vi "Read Session.vi"(8 "error in":errorcluster, 11 "Fgen PXI in":refnum<class "Fgen PXI.lvclass">) -> (0 "error out":errorcluster, 2 "Session":refnum<k15>, 3 "Fgen PXI out":refnum<class "Fgen PXI.lvclass">)   [LabVIEW 2023, in "Fgen PXI.lvlib" / "Fgen PXI.lvclass"]
uses:
  Fgen PXI.lvclass
  Fgen PXI.lvclass/Fgen PXI.ctl
  Fgen PXI CFG/Fgen PXI CFG.lvclass
  D:/git/HAL/Fgen Base/Fgen Base.lvclass
  D:/git/HAL/Instrument/Instrument.lvclass
  D:/git/HAL/Interfaces/IFGEN/IFGEN.lvclass
  D:/git/HAL/Fgen PXI/Fgen PXI.lvclass
  Fgen Base/Fgen Base.lvclass
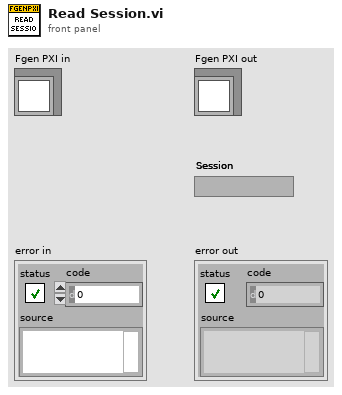
[diagram p1: front panel]
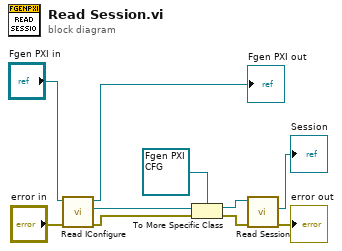
[diagram p0: block diagram]
diagram:
  n1 = call "Read IConfigure.vi"("error in (no error)"="error in", "Fgen Base in"="Fgen PXI in") -> ("error out"=w3:errorcluster, "IConfigure"=w4:refnum<class "IConfigure.lvclass">, "Fgen Base out"=→"Fgen PXI out":refnum<class "Fgen PXI.lvclass">)  [unwired: 7 in]
  n2 = To More Specific Class(target class=refnum<class "Fgen PXI CFG.lvclass"> refnum ("Fgen PXI.lvlib:Fgen PXI CFG.lvclass"), reference=w4, error in=w3) -> (specific class reference=w1:refnum<class "Fgen PXI CFG.lvclass">, error out=w2:errorcluster)
  n3 = call "Read Session.vi"("error in (no error)"=w2, "Fgen PXI CFG in"=w1) -> ("error out"=→"error out":errorcluster, "Session"=→"Session":refnum<k15>)  [unwired: 7 in, 1 out]
